vi "Preserve Run-Time Class.vi"() -> ()   [LabVIEW 2023]
doc: "This example shows two ways to preserve the object type when passing classes through subVIs. In one case the same object propagates from the input to the output of the subVI. In the other case, the new Preserve Run-Time Class function is used."
uses:
  Child/Child.lvclass
  c:/dev/_r/4/eng/lv-core/lvpostprocessingd/lv_mc_x86_64/dist_i386/examples/Object-Oriented Programming/Preserve Run-Time Class/Parent/Parent.lvclass
  Parent/Parent.lvclass
panel:
  out "Child 4":refnum<class "Child.lvclass">
  out "Child 3":refnum<class "Child.lvclass">
  out "Child 2":refnum<class "Child.lvclass">
  out "Child 1":refnum<class "Child.lvclass">
  # "Overview: This example shows how to preserve the object type when passing classes through subVIs, by using the Preserve Run-Time Class function.\nInstructions:\n1. Open the block diagram and refer to the comments there.\n2. You do not need to run this VI."
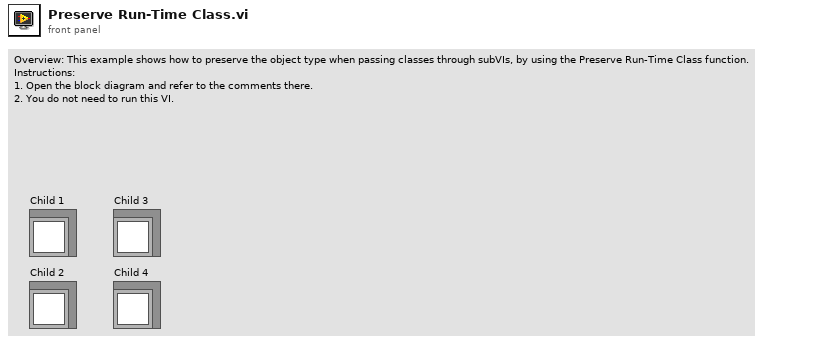
[diagram p1: front panel]
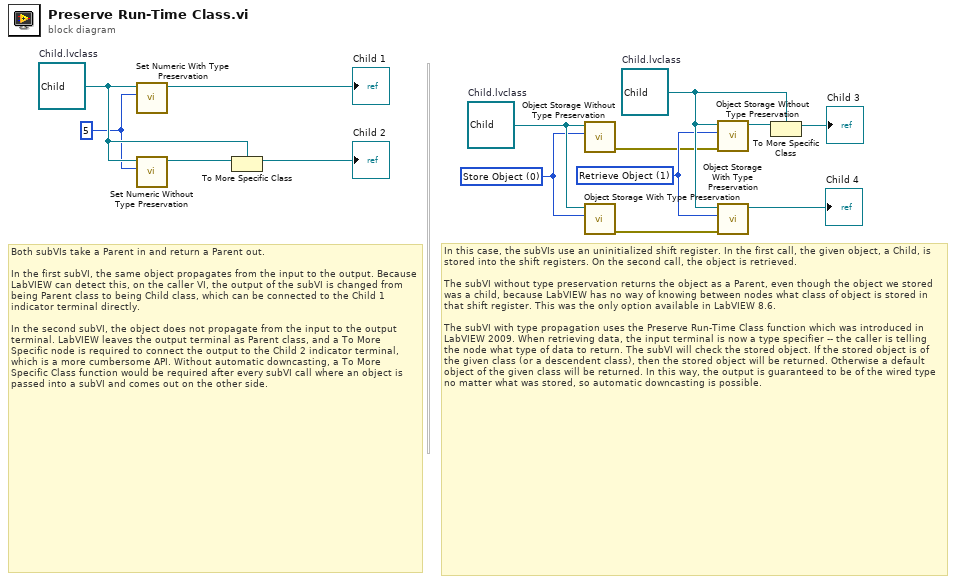
[diagram p0: block diagram]
diagram:
  w4 = u16 1 items=["Store Object", "Retrieve Object"] ("Action")
  w5 = refnum<class "Child.lvclass"> refnum  # Child.lvclass
  w6 = u16 0 items=["Store Object", "Retrieve Object"] ("Action")
  w7 = refnum<class "Child.lvclass"> refnum  # Child.lvclass
  w10 = 5 ("Numeric")
  w12 = refnum<class "Child.lvclass"> refnum  # Child.lvclass
  # "In this case, the subVIs use an uninitialized shift register. In the first call, the given object, a Child, is stored into the shift registers. On the second call, the object is retrieved.\n\nThe subVI without type preservation returns the object as a Parent, even though the object we stored was a child, because LabVIEW has no way of knowing between nodes what class of object is stored in that shift register. This was the only option available in LabVIEW 8.6.\n\nThe subVI with type propagation uses the Preserve Run-Time Class function which was introduced in LabVIEW 2009. When retrieving data, the input terminal is now a type specifier -- the caller is telling the node what type of data to return. The subVI will check the stored object. If the stored object is of the given class (or a descendent class), then the stored object will be returned. Otherwise a default object of the given class will be returned. In this way, the output is guaranteed to be of the wired type no matter what was stored, so automatic downcasting is possible."
  # "Both subVIs take a Parent in and return a Parent out.\n\nIn the first subVI, the same object propagates from the input to the output. Because LabVIEW can detect this, on the caller VI, the output of the subVI is changed from being Parent class to being Child class, which can be connected to the Child 1 indicator terminal directly.\n\nIn the second subVI, the object does not propagate from the input to the output terminal. LabVIEW leaves the output terminal as Parent class, and a To More Specific node is required to connect the output to the Child 2 indicator terminal, which is a more cumbersome API. Without automatic downcasting, a To More Specific Class function would be required after every subVI call where an object is passed into a subVI and comes out on the other side."
  n1 = call "Set Numeric With Type Preservation.vi"("Numeric"=w10, "Parent in"=w12) -> ("Parent out"=→"Child 1":refnum<class "Child.lvclass">)  [unwired: 9 out]
  n2 = call "Set Numeric Without Type Preservation.vi"("Numeric"=w10, "Parent in"=w12) -> ("Parent out"=w13:refnum<class "Parent.lvclass">)  [unwired: 9 out]
  n3 = To More Specific Class(target class=w12, reference=w13) -> (specific class reference=→"Child 2":refnum<class "Child.lvclass">)  [unwired: 1 in, 1 out]
  n4 = call "Object Storage Without Type Preservation.vi"("Action"=w6, "Object in"=w7) -> ("error out"=w3:errorcluster)  [unwired: 8 in, 1 out]
  n5 = call "Object Storage With Type Preservation.vi"("Action"=w6, "Object in"=w7) -> ("error out"=w9:errorcluster)  [unwired: 8 in, 1 out]
  n6 = call "Object Storage Without Type Preservation.vi"("error in (no error)"=w3, "Action"=w4, "Object in"=w5) -> ("Object out"=w2:refnum<class "Parent.lvclass">)  [unwired: 7 in, 1 out]
  n7 = call "Object Storage With Type Preservation.vi"("error in (no error)"=w9, "Action"=w4, "Object in"=w5) -> ("Object out"=→"Child 4":refnum<class "Child.lvclass">)  [unwired: 7 in, 1 out]
  n8 = To More Specific Class(target class=w5, reference=w2) -> (specific class reference=→"Child 3":refnum<class "Child.lvclass">)  [unwired: 1 in, 1 out]
